vi "Open Front Panel.vi"(8 "error in (no error)":errorcluster, 11 "Meter Measurement in":refnum<class "Meter Measurement.lvclass">) -> (0 "error out":errorcluster, 3 "Meter Measurement out":refnum<class "Meter Measurement.lvclass">)   [LabVIEW 2015, in "Meter Measurement.lvclass"]
uses:
  Meter Measurement.lvclass
  Meter Measurement.lvclass/Meter Measurement.ctl
  <vilib>/ActorFramework/Message Enqueuer/Message Enqueuer.lvclass/Message Enqueuer.ctl
  <vilib>/ActorFramework/Message Enqueuer/Enqueue.vi
  <vilib>/ActorFramework/Message Priority Queue/Priority Enqueue.vi
  Mag Lab Root Messages/Open Front Panel Msg/Open Front Panel Msg.lvclass
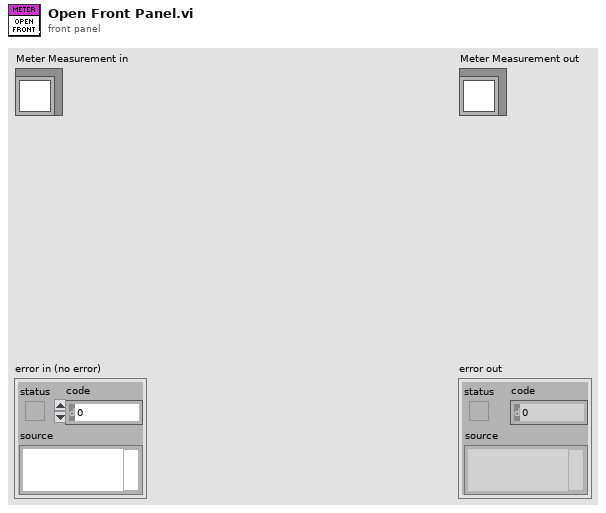
[diagram p1: front panel]
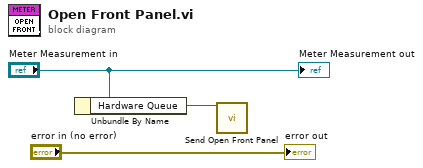
[diagram p0: block diagram]
diagram:
  n1 = Unbundle By Name("Meter Measurement in") -> ("Hardware Queue"=w3:refnum<class "Message Enqueuer.lvclass">)
  n2 = call "Send Open Front Panel.vi"("Message Enqueuer"=w3) -> ()  [unwired: 9 in, 2 out]
  "error out" <- "error in (no error)"
  "Meter Measurement out" <- "Meter Measurement in"
